vi "Read File and Remove Header.vi"(8 "error in (no error)":errorcluster, 11 "selected path":path) -> (0 "error out":errorcluster, 3 "Array":string[](array[string]))   [LabVIEW 2019, in "Diagnostics Addon System Explorer.lvlib"]
uses:
  Diagnostics Addon System Explorer.lvlib
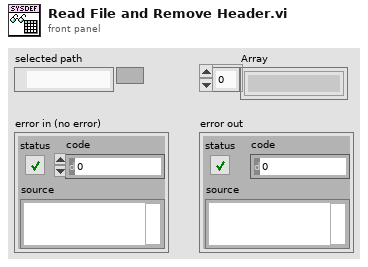
[diagram p1: front panel]
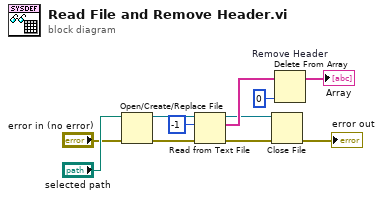
[diagram p0: block diagram]
diagram:
  n1 = Open/Create/Replace File(file path (use dialog)="selected path", error in="error in (no error)") -> (refnum out=w2:refnum<file>, error out=w1:errorcluster)  [unwired: 4 in, 1 out]
  n2 = Read from Text File(file (use dialog)=w2, count=-1, error in=w1) -> (refnum out=w3:refnum<file>, text=w9:string[], error out=w4:errorcluster)  [unwired: 1 in, 1 out]
  n3 = Close File(refnum=w3, error in=w4) -> (error out=→"error out":errorcluster)  [unwired: 1 out]
  n4 = Delete From Array "Remove Header"(array=w9, index=0) -> (array with subset deleted=→"Array":string[])  [unwired: 1 in, 1 out]
